vi "MOCR.vi"() -> ()   [LabVIEW 2020]
uses:
  Typedefs/MOCR-State.ctl
  Typedefs/MOCR-Parameters.ctl
panel:
  in  "Options":bool
  in  "result":T1
  out "Progress":u8(slide) scale=0.0..10.0
  in  "Property":dbl
  in  "Channel":string
  in  "Start":bool
  in  "Stop":bool
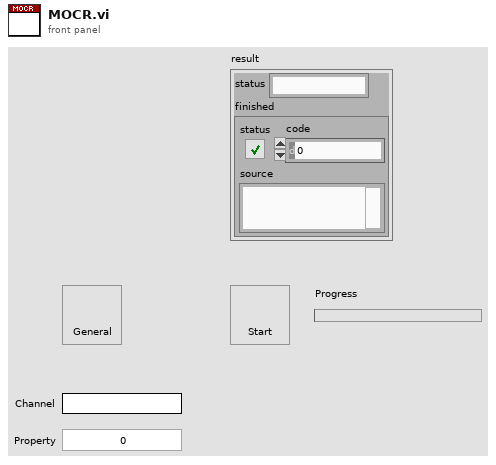
[diagram p1: front panel]
types:
  T1 = cluster{"status":string, "finished":errorcluster}
  T2 = typedef "MOCR-Parameters.ctl" = cluster{"Channel":string, "Property":dbl}
  T3 = typedef "MOCR-State.ctl" = cluster{"running":bool}
  T4 = enum8{"Enabled", "Disabled", "Disabled and Grayed Out"}
  T5 = cluster{string, "\"Settings\" or \"Parameters\"":T2}
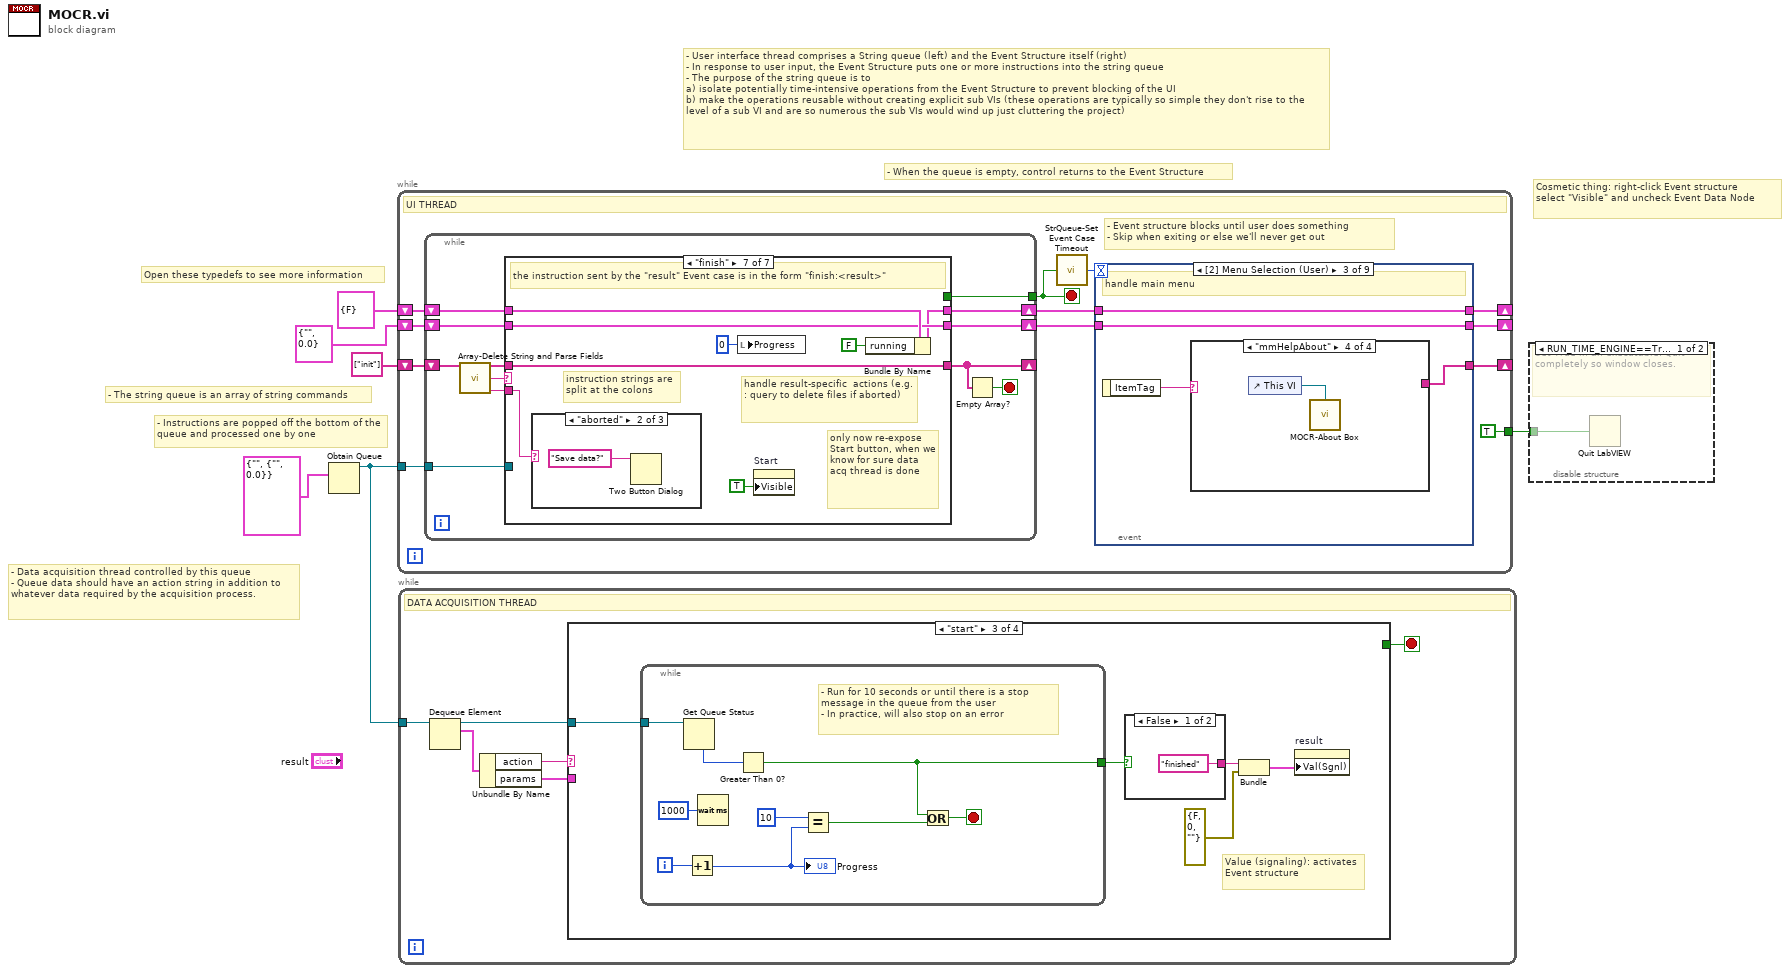
[diagram p0: block diagram]
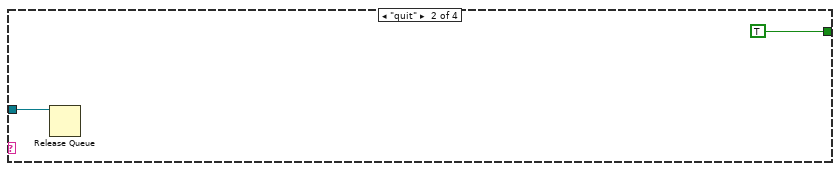
[diagram p3: hidden frame]
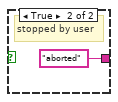
[diagram p4: hidden frame]
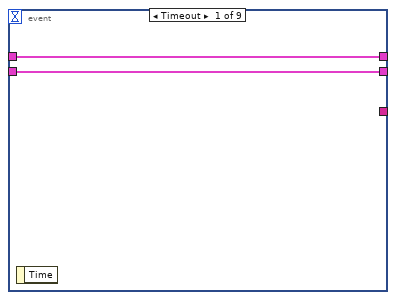
[diagram p6: hidden frame]
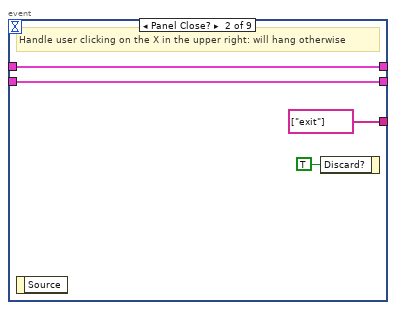
[diagram p7: hidden frame]
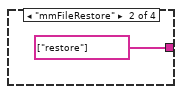
[diagram p9: hidden frame]
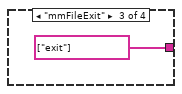
[diagram p10: hidden frame]
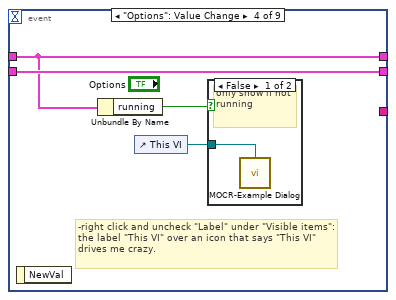
[diagram p11: hidden frame]
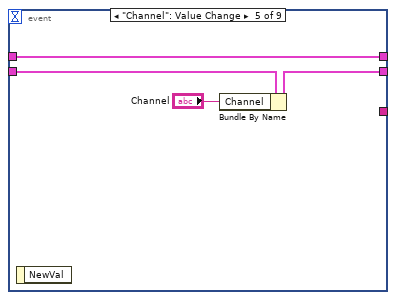
[diagram p13: hidden frame]
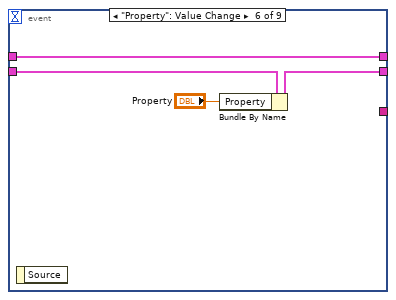
[diagram p14: hidden frame]
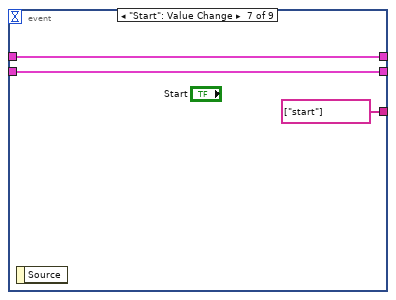
[diagram p15: hidden frame]
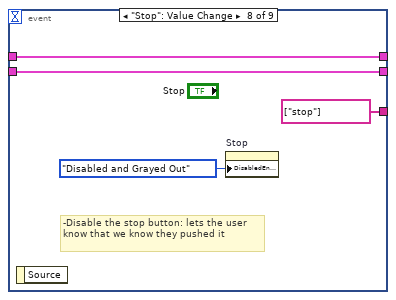
[diagram p16: hidden frame]
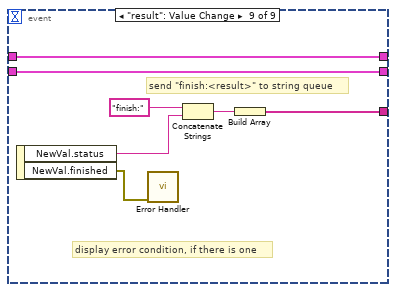
[diagram p17: hidden frame]
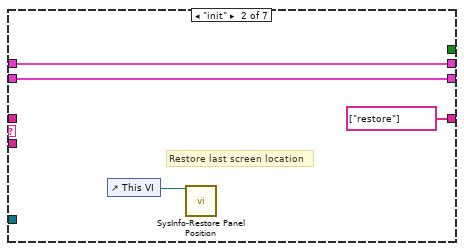
[diagram p19: hidden frame]
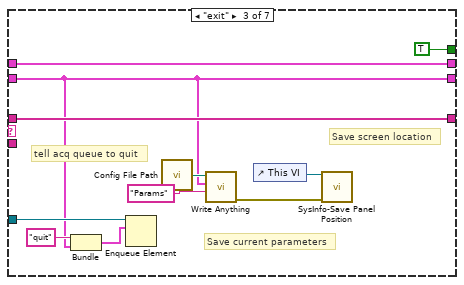
[diagram p20: hidden frame]
diagram:
  # "- Data acquisition thread controlled by this queue\n- Queue data should have an action string in addition to whatever data required by the acquisition process."
  # "Cosmetic thing: right-click Event structure\nselect \"Visible\" and uncheck Event Data Node"
  # "Open these typedefs to see more information"
  # "- Instructions are popped off the bottom of the queue and processed one by one"
  # "- When the queue is empty, control returns to the Event Structure"
  # "- The string queue is an array of string commands"
  # "- User interface thread comprises a String queue (left) and the Event Structure itself (right)\n- In response to user input, the Event Structure puts one or more instructions into the string queue\n- The purpose of the string queue is to \na) isolate potentially time-intensive operations from the Event Structure to prevent blocking of the UI\nb) make the operations reusable without creating explicit sub VIs (these operations are typically so simple they don't rise to the level of a sub VI and are so numerous the sub VIs would wind up just cluttering the project)"
  n1 = Obtain Queue(element data type=cluster{"action":string, "params":T2} {"action"="", "params"={"Channel"="", "Property"=0.0}}) -> (queue out=w2:refnum<queue>)  [unwired: 4 in, 2 out]
  n2 = while {
    shift-right: [w15] -> _
    shift-left: string[] ["init"] -> [w16]
    shift-right: [w12] -> _
    shift-left: T3 {"running"=FALSE} ("State") -> [w14]
    shift-right: [w9] -> _
    shift-left: T2 {"Channel"="", "Property"=0.0} ("\"Settings\" or \"Parameters\"") -> [w11]
    tunnel: [TRUE] -> w3
    tunnel: w2 -> [w7]
    stop <- w18 stop-if-true
    # "- Event structure blocks until user does something\n- Skip when exiting or else we'll never get out"
    # "UI THREAD"
    n3 = while {
      shift-right: [w70] -> _
      shift-left: w16 -> [w67]
      tunnel: [w68] -> w18
      shift-right: [w63] -> w13
      shift-left: w14 -> [w64]
      shift-right: [w61] -> w10
      shift-left: w11 -> [w62]
      tunnel: w7 -> [w60]
      stop <- w69 stop-if-true
      n4 = call "Array-Delete String and Parse Fields.vi"("Array in"=w67) -> ("Array out"=w66:string[], "Field 1"=w65:string, "Field 2"=w59:string)  [unwired: 10 in, 2 out]
      n5 = case shown="\"finish\"" w65 {
        tunnel: w66 -> [w73 _ w88 w99 w114 w120 w128]
        tunnel: [w73 string[] ["restore"] ("Array out") w88 w99 w114 w120 w128] -> w70
        tunnel: [_ _ TRUE _ _ _ _] -> w68
        tunnel: w64 -> [w72 w77 w86 w98 w113 w119 w127]
        tunnel: [w72 w77 w86 w98 w106 w119 w123] -> w63
        tunnel: w62 -> [w71 w76 w79 w94 w109 w115 w126]
        tunnel: [w71 w76 w79 w91 w109 w115 w126] -> w61
        tunnel: w60 -> [_ _ w81 _ w110 w116 _]
        tunnel: w59 -> [_ _ _ _ _ _ w125]
        frame "", Default {
        }
        frame "init" {
          # "Restore last screen location"
          n6 = control-ref of="This VI"() -> (w75:refnum<vi>)
          n7 = call "SysInfo-Restore Panel Position.vi"("VI Refnum"=w75) -> ()  [unwired: 12 in, 3 out]
        }
        frame "exit" {
          # "tell acq queue to quit"
          # "Save current parameters"
          # "Save screen location"
          n8 = Bundle("quit", "\"Settings\" or \"Parameters\""=w79) -> (w78:T5)  [unwired: 1 in]
          n9 = Enqueue Element(queue=w81, element=w78) -> ()  [unwired: 2 in, 3 out]
          n10 = call "Config File Path.vi"() -> ("Default config file name"=w83:path)  [unwired: 1 in]
          n11 = call "Write Anything.vi"("Section Name (Name of \"Anything\")"="Params" ("Section Name (Name of \"Anything\")"), "Anything"=w79, "Path (dialog)"=w83) -> ("Error Out"=w84:errorcluster)  [unwired: 7 in, 1 out]
          n12 = control-ref of="This VI"() -> (w85:refnum<vi>)
          n13 = call "SysInfo-Save Panel Position.vi"("VI Refnum"=w85, "error in (no error)"=w84) -> ()  [unwired: 13 in, 1 out]
        }
        frame "restore" {
          # "Restore parameters"
          n14 = call "Config File Path.vi"() -> ("Default config file name"=w97:path)  [unwired: 1 in]
          n15 = call "Read Anything.vi"("Type of Anything"=w94, "Section Name (Name of \"Type of Anything\")"="Params" ("Section Name (Name of \"Type of Anything\")"), "Path (dialog)"=w97) -> ("Error Out"=w92:errorcluster, "Found?"=w93:bool, "Anything"=w95:variant)  [unwired: 6 in]
          n16 = case shown="True" w93 {
            tunnel: w95 -> [_ w103]
            tunnel: w94 -> [w100 w102]
            tunnel: w92 -> [_ w104]
            tunnel: [w100 w101] -> w91
            frame False {
            }
            frame True {
              n17 = Variant To Data(error in=w104, type=w102, Variant=w103) -> (data=w101:T2)  [unwired: 1 out]
            }
          }
          n18 = Unbundle By Name(w91) -> ("Channel"=w90:string, "Property"=w89:dbl)
          n19 = local write "Channel"(w90) -> ()
          n20 = local write "Property"(w89) -> ()
        }
        frame "start" {
          # "Make sure Stop is enabled"
          # "Hide the Start (exposing Stop)"
          n21 = Bundle("start", "\"Settings\" or \"Parameters\""=w109) -> (w111:T5)  [unwired: 1 in]
          n22 = Enqueue Element(queue=w110, element=w111) -> ()  [unwired: 2 in, 3 out]
          n23 = property on="Stop" class="Bool"("DisabledEnum"=T4."Enabled" ("Disabled")) -> ()  [unwired: 2 in, 2 out]
          n24 = property on="Start" class="Bool"("Visible"=FALSE) -> ()  [unwired: 2 in, 2 out]
          n25 = Bundle By Name(cluster=w113, "running"=TRUE) -> (w106:T3)
        }
        frame "stop" {
          n26 = Bundle("stop", "\"Settings\" or \"Parameters\""=w115) -> (w117:T5)  [unwired: 1 in]
          n27 = Enqueue Element(queue=w116, element=w117) -> ()  [unwired: 2 in, 3 out]
        }
        frame "finish" {
          # "only now re-expose Start button, when we know for sure data acq thread is done"
          # "handle result-specific  actions (e.g.: query to delete files if aborted)"
          # "instruction strings are split at the colons"
          # "the instruction sent by the \"result\" Event case is in the form \"finish:<result>\""
          n28 = case shown="\"aborted\"" w125 {
            frame "", Default {
            }
            frame "aborted" {
              n29 = Two Button Dialog(message="Save data?") -> ()  [unwired: 2 in, 1 out]
            }
            frame "finished" {
            }
          }
          n30 = local write "Progress"(u8 0 ("Progress")) -> ()
          n31 = property on="Start" class="Bool"("Visible"=TRUE) -> ()  [unwired: 2 in, 2 out]
          n32 = Bundle By Name(cluster=w127, "running"=FALSE) -> (w123:T3)
        }
      }
      n33 = Empty Array?(array=w70) -> (empty?=w69:bool)
    }
    n34 = call "StrQueue-Set Event Case Timeout.vi"("Quit"=w18) -> ("timeout"=w17:i32)  [unwired: 14 in]
    n35 = event shown="[2] Menu Selection (User)" {
      selector: _ -> [_ _ _ _ _ _ _ _ _]
      dyn-events: _ -> [_ _ _ _ _ _ _ _ _]
      timeout: w17 -> [_ _ _ _ _ _ _ _ _]
      tunnel: [_ string[] ["exit"] w25 _ _ _ string[] ["start"] string[] ["stop"] w52] -> w15
      tunnel: w13 -> [w20 w22 w28 w33 w40 w44 w47 w51 w58]
      tunnel: [w20 w22 w28 w33 w40 w44 w47 w51 w58] -> w12
      tunnel: w10 -> [w19 w21 w27 w35 w39 w43 w46 w50 w57]
      tunnel: [w19 w21 w27 w35 w38 w42 w46 w50 w57] -> w9
      event Timeout {
        n36 = event-data() -> ()  [unwired: 1 in, 1 out]
      }
      event Panel Close? {
        # "Handle user clicking on the X in the upper right: will hang otherwise"
        n37 = event-data() -> ()  [unwired: 1 in, 1 out]
        n38 = event-data("Discard?"=TRUE) -> ()  [unwired: 1 in, 1 out]
      }
      event Menu Selection (User) {
        # "handle main menu"
        n39 = event-data() -> ("ItemTag"=w26:string)  [unwired: 1 in]
        n40 = case shown="\"mmHelpAbout\"" w26 {
          tunnel: [_ string[] ["restore"] string[] ["exit"] _] -> w25
          frame "", Default {
          }
          frame "mmFileRestore" {
          }
          frame "mmFileExit" {
          }
          frame "mmHelpAbout" {
            n41 = control-ref of="This VI"() -> (w31:refnum<vi>)
            n42 = call "MOCR-About Box.vi"("Parent VI"=w31) -> ()  [unwired: 15 in]
          }
        }
      }
      event "Options": Value Change {
        # "-right click and uncheck \"Label\" under \"Visible items\": the label \"This VI\" over an icon that says \"This VI\" drives me crazy."
        n43 = event-data() -> ()  [unwired: 1 in, 1 out]
        n44 = Unbundle By Name(w33) -> ("running"=w32:bool)
        n45 = control-ref of="This VI"() -> (w34:refnum<vi>)
        n46 = case shown="False" w32 {
          tunnel: w34 -> [w36 _]
          frame False {
            # "only show if not running"
            n47 = call "MOCR-Example Dialog.vi"("Parent VI"=w36) -> ()  [unwired: 13 in, 2 out]
          }
          frame True {
          }
        }
      }
      event "Channel": Value Change {
        n48 = event-data() -> ()  [unwired: 1 in, 1 out]
        n49 = Bundle By Name(cluster=w39, "Channel"="Channel") -> (w38:T2)
      }
      event "Property": Value Change {
        n50 = event-data() -> ()  [unwired: 1 in, 1 out]
        n51 = Bundle By Name(cluster=w43, "Property"="Property") -> (w42:T2)
      }
      event "Start": Value Change {
        n52 = event-data() -> ()  [unwired: 1 in, 1 out]
      }
      event "Stop": Value Change {
        # "-Disable the stop button: lets the user know that we know they pushed it"
        n53 = event-data() -> ()  [unwired: 1 in, 1 out]
        n54 = property on="Stop" class="Bool"("DisabledEnum"=T4."Disabled and Grayed Out" ("Disabled")) -> ()  [unwired: 2 in, 2 out]
      }
      event "result": Value Change {
        # "send \"finish:<result>\" to string queue"
        # "display error condition, if there is one"
        n55 = event-data() -> ("NewVal.status"=w55:string, "NewVal.finished"=w54:errorcluster)  [unwired: 1 in]
        n56 = call "Error Handler.vi"("error in (no error)"=w54) -> ()  [unwired: 12 in, 3 out]
        n57 = Concatenate Strings("finish:" ("string"), w55) -> (w53:string)
        n58 = Build Array(w53) -> (w52:string[])
      }
    }
  }
  n59 = while {
    tunnel: w2 -> [w135]
    stop <- w132 stop-if-true
    # "DATA ACQUISITION THREAD"
    n60 = Dequeue Element(queue=w135) -> (queue out=w130:refnum<queue>, element=w131:cluster{"action":string, "params":T2})  [unwired: 2 in, 2 out]
    n61 = Unbundle By Name(w131) -> ("action"=w134:string, "params"=w133:T2)
    n62 = case shown="\"start\"" w134 {
      tunnel: w133 -> [_ _ _ _]
      tunnel: [_ TRUE _ _] -> w132
      tunnel: w130 -> [_ w136 w142 _]
      frame "", Default {
      }
      frame "quit" {
        n63 = Release Queue(queue=w136) -> ()  [unwired: 2 in, 3 out]
      }
      frame "start" {
        # "Value (signaling): activates Event structure"
        n64 = while {
          tunnel: w142 -> [w153]
          tunnel: [w145] -> w141
          i -> [w150]
          stop <- w147 stop-if-true
          # "- Run for 10 seconds or until there is a stop message in the queue from the user\n- In practice, will also stop on an error"
          n65 = Get Queue Status(queue=w153) -> (# elements in queue=w152:i32)  [unwired: 2 in, 7 out]
          n66 = Increment(x=w150) -> (x+1=w149:i32)
          "Progress" <- w149
          n67 = Wait (ms)(milliseconds to wait=u32 1000) -> ()  [unwired: 1 out]
          n68 = Greater Than 0?(x=w152) -> (x > 0?=w145:bool)
          n69 = Equal?(x=10, y=w149) -> (x = y?=w146:bool)
          n70 = Or(x=w145, y=w146) -> (x .or. y?=w147:bool)
        }
        n71 = case shown="False" w141 {
          tunnel: ["finished" "aborted"] -> w140
          frame False {
          }
          frame True {
            # "stopped by user"
          }
        }
        n72 = Bundle(w140, "error constant"=errorcluster {"status"=FALSE, "code"=0, "source"=""}) -> (w138:cluster{string, "error constant":errorcluster})  [unwired: 1 in]
        n73 = property on="result" class="Clust (strict)"("Val(Sgnl)"=w138) -> ()  [unwired: 2 in, 2 out]
      }
      frame "stop" {
      }
    }
  }
  n74 = disable-structure shown="RUN_TIME_ENGINE==True" {
    disable-tunnel: w3 -> [w154 _]
    frame condition #0 {
      # "Set True in an executable. Quit completely so window closes."
      n75 = Quit LabVIEW(quit? (T)=w154) -> ()
    }
    frame condition #1 (active) {
      # "Running in LabVIEW development system. Leaves window open"
    }
  }
